vi "Joystick Plugin Ref.vi"() -> (1 "Command Index":cluster{i32, i32}, 2 "Plugin VI Ref":refnum<vi>, 3 "Device Type":string)   [LabVIEW 2019]
uses:
  Joystick Update Ops.ctl
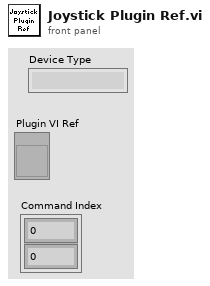
[diagram p1: front panel]
types:
  T1 = typedef "Joystick Update Ops.ctl" = enum16{"set init", "set buttons", "set povs", "set axes", "set left_rumble", "set right_rumble", "set outputs", "get", "delete", "JSON update", "set name", "transmit initial", "reset"}
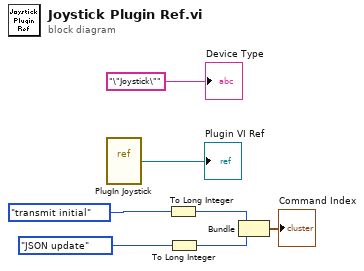
[diagram p0: block diagram]
diagram:
  n1 = vi-ref "PlugIn Joystick.vi"() -> (→"Plugin VI Ref":refnum<vi>)
  n2 = To Long Integer(number=Joystick_Update_Ops."transmit initial" ("menu")) -> (32bit integer=w4:i32)
  n3 = To Long Integer(number=Joystick_Update_Ops."JSON update" ("menu")) -> (32bit integer=w3:i32)
  n4 = Bundle(w4, w3) -> (→"Command Index":cluster{i32, i32})  [unwired: 1 in]
  "Device Type" <- "\"Joystick\""
